vi "FindRequiredComponents2.vi"(4 "Version Selection Modes":u32[](array[numeric]), 5 "Software IDs to Uninstall":string[](array[string]), 6 "Software to Install":T1[](array[typedef]) {"component type" items=["standard", "hidden", "system", "unknown", "startup", "image", "essential"]}, 7 "Item Types (all visible)":T4 items=["all visible", "all including hidden", "standard only", "startup only"], 8 "error in (no error)":errorcluster, 9 "Component Version":string, 10 "Component ID":string, 11 "Session in":refnum<k21>) -> (0 "error out":errorcluster, 2 "Required Components":T3[](array[typedef]) {"Visibility Type" items=["standard", "hidden", "system", "unknown", "startup", "image", "essential"]}, 3 "Session out":refnum<k21>)   [LabVIEW 2017, in "nisyscfg.lvlib"]
uses:
  <vilib>/nisyscfg/nisyscfg.lvlib
  <vilib>/nisyscfg/Component Types.ctl
  <vilib>/nisyscfg/Software Extended.ctl
  <vilib>/nisyscfg/Component Type.ctl
  <vilib>/nisyscfg/Software 1.2.ctl
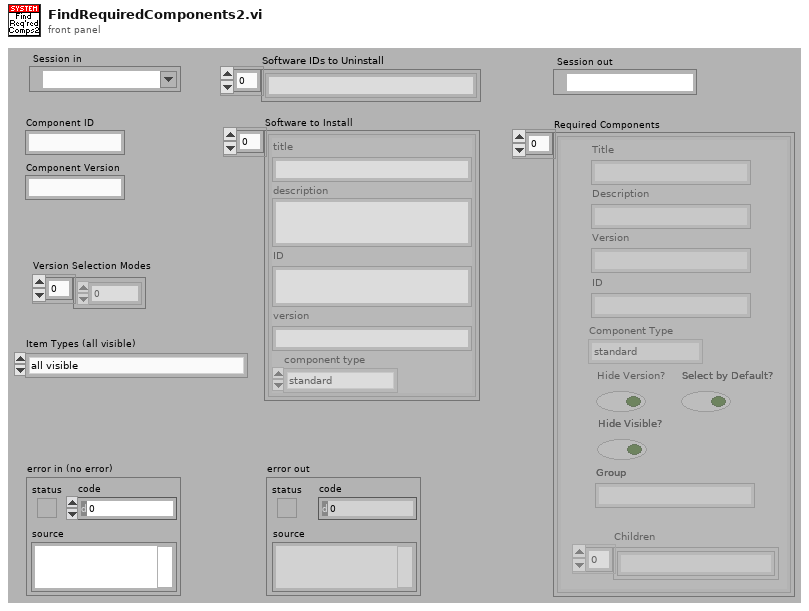
[diagram p1: front panel]
types:
  T1 = typedef "nisyscfg.lvlib/Software 1.2.ctl" = cluster{"title":string, "description":string, "ID":string, "version":string, "component type":T2}
  T2 = typedef "nisyscfg.lvlib/Component Type.ctl" = u32
  T3 = typedef "nisyscfg.lvlib/Software Extended.ctl" = cluster{"Description":string, "ID":string, "Version":string, "Title":string, "Visibility Type":T2, "Hide Version?":bool, "Children":string[], "Select by Default?":bool, "Hide Visible?":bool, "Group":string}
  T4 = typedef "nisyscfg.lvlib/Component Types.ctl" = u32
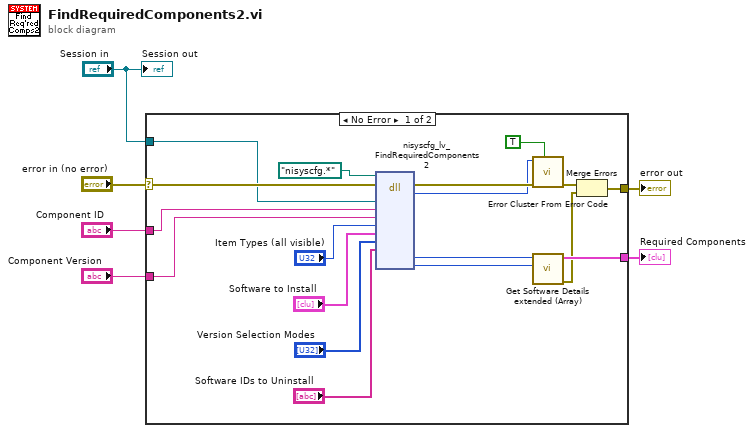
[diagram p0: block diagram]
diagram:
  n1 = case shown="No Error" "error in (no error)" {
    selector: "error in (no error)" -> [w22 w25]
    tunnel: "Session in" -> [w21 _]
    tunnel: "Component Version" -> [w19 _]
    tunnel: "Component ID" -> [w18 _]
    tunnel: [w12 w25] -> w2
    tunnel: [w16 _] -> w1
    frame No Error {
      n2 = dll-call lib="nisyscfg.*" fn="nisyscfg_lv_FindRequiredComponents2" label="FindRequiredComponents2"(path in=path "nisyscfg.*", error in=w22, "session"=w21, "componentID"=w18, "componentVersion"=w19, "includeTypes"="Item Types (all visible)", "softwareToInstall"="Software to Install", "versionSelectionModes"="Version Selection Modes", "softwareIDsToUninstall"="Software IDs to Uninstall") -> (error out=w24:errorcluster, "result"=w23:i32, "requiredComponents"=w15:u64, "numComponents"=w11:i32)  [unwired: 10 in, 1 out]
      n3 = call <vilib>:"Error Cluster From Error Code.vi"("show call chain? (False)"=TRUE, "error in (no error)"=w24, "error code (0)"=w23) -> ("error out"=w14:errorcluster)  [unwired: 6 in]
      n4 = call <vilib>:"Get Software Details extended (Array).vi"("Number of Elements"=w11, "Enumerator in"=w15) -> ("error out"=w13:errorcluster, "Software Components"=w16:T3[])  [unwired: 8 in]
      n5 = Merge Errors(w14, w13) -> (w12:errorcluster)
    }
    frame Error {
    }
  }
  "error out" <- w2
  "Required Components" <- w1
  "Session out" <- "Session in"
